vi "read_matrices.vi"() -> (0 "Matrix Matlab":T1)   [LabVIEW 2021]
uses:
  <vilib>/Analysis/Matrix/Datatypes/RealMatrix.ctl
  <vilib>/Utility/xml.llb/Read From XML File(string).vi
  <vilib>/Analysis/Matrix/NI_Matrix.lvlib
panel:
  in  "Real Matrix":T1
  in  "XML File Path load matrix":path=path "c:/ni-rt/startup/matrixmat.xml"
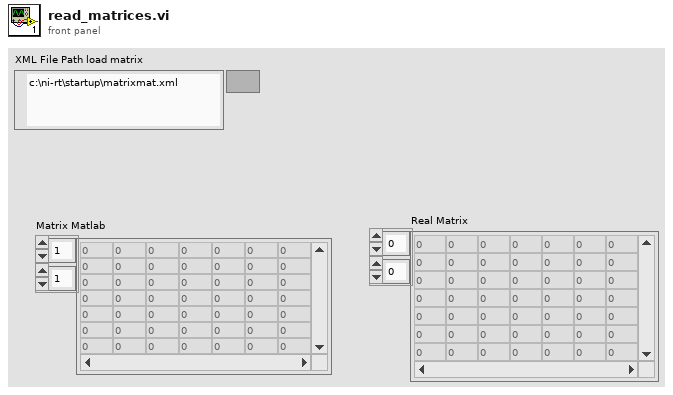
[diagram p1: front panel]
types:
  T1 = typedef "NI_Matrix.lvlib/RealMatrix.ctl" = dbl[][]
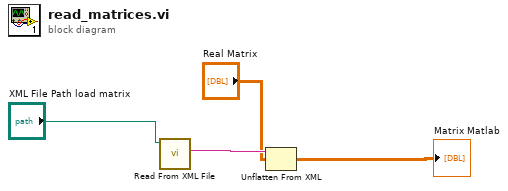
[diagram p0: block diagram]
diagram:
  n1 = call-poly <vilib>:"Read From XML File.vi"("XML File Path"="XML File Path load matrix") -> ("XML Elements"=w4:string)  [unwired: 8 in, 2 out]
  n2 = Unflatten From XML(xml string=w4, type="Real Matrix") -> (value=→"Matrix Matlab":T1)  [unwired: 1 in, 1 out]
